vi "CheckForNI6629.vi"   [LabVIEW 2009]
uses:
  H:/Program Files/National Instruments/LabVIEW 2009/resource/objmgr/daqmx.rc
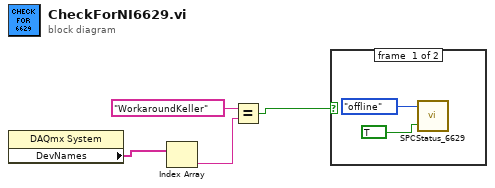
[diagram p0: block diagram]
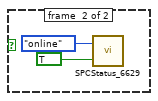
[diagram p2: hidden frame]
diagram:
  n1 = property class="DAQmx System"() -> ("DevNames"=w1:tag[])  [unwired: 2 in, 2 out]
  n2 = Index Array(array=w1) -> (element=w4:tag)  [unwired: 1 in]
  n3 = Equal?(x=tag "WorkaroundKeller", y=w4) -> (x = y?=w2:bool)
  n4 = case shown="True" w2 {
    frame #0 {
      n5 = call "SPCStatus_6629.vi"("Set/Get"=TRUE, "Status (input)"=enum16{"offline", "online", "busy"}."offline") -> ()  [unwired: 1 out]
    }
    frame #1 {
      n6 = call "SPCStatus_6629.vi"("Set/Get"=TRUE, "Status (input)"=enum16{"offline", "online", "busy"}."online") -> ()  [unwired: 1 out]
    }
  }
